vi "get channels test.vi"() -> (0 "error out":errorcluster, 3 "channels match":bool)   [LabVIEW 2014, in "UI Reference tests.lvlib"]
doc: "Tests the 'Get Channels' VI of the Configuration class."
uses:
  UI Reference tests.lvlib
  module/configuration/UI Reference configuration.lvclass
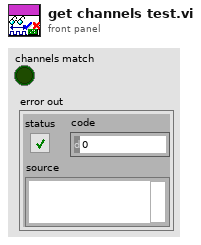
[diagram p1: front panel]
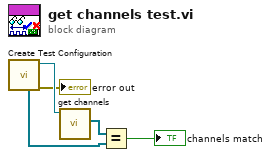
[diagram p0: block diagram]
diagram:
  n1 = call "Create Test Configuration.vi"() -> ("error out"=→"error out":errorcluster, "Module Configuration"=w5:refnum<class "UI Reference configuration.lvclass">, "Channels"=w2:refnum<class "TBM channel.lvclass">[])  [unwired: 6 in, 3 out]
  n2 = call-dynamic "get channels.vi"("UI Reference configuration in"=w5) -> ("channels"=w3:refnum<class "TBM channel.lvclass">[])  [unwired: 9 in, 1 out]
  n3 = Equal?(x=w3, y=w2) -> (x = y?=→"channels match":bool)
